vi "testControlNotOnConnectorPane.vi"() -> ()   [LabVIEW 2019, in "TestCaseTest.lvlib" / "Theory.lvlib"]
uses:
  Theory.lvlib
  TestCase/Theory/Theory.lvclass
  TestCaseTestSupport/FakeTheoryWithControlsNotOnConnectorPane.vi
  Assertion/Assertion.lvlib
  TestCaseTestSupport/TestCaseTestSupport.lvlib
panel:
  out "error out":errorcluster
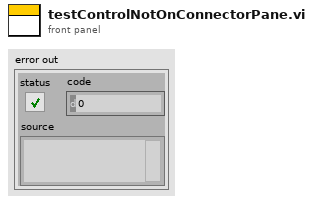
[diagram p1: front panel]
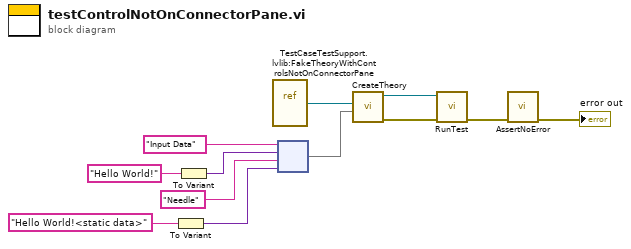
[diagram p0: block diagram]
diagram:
  n1 = To Variant(anything="Hello World!<static data>" ("key")) -> (Variant=w2:variant)
  n2 = To Variant(anything="Hello World!" ("key")) -> (Variant=w6:variant)
  n3 = vi-ref "TestCaseTestSupport.lvlib:FakeTheoryWithControlsNotOnConnectorPane.vi"() -> (w4:refnum<vi>)
  n4 = node("Input Data" ("key"), w6, "Needle" ("key"), w2) -> (w7:map{string, variant})
  n5 = call "CreateTheory.vi"("Control Data"=w7, "VI Refnum"=w4) -> ("error out"=w11:errorcluster, "Theory"=w12:refnum<class "Theory.lvclass">)  [unwired: 8 in]
  n6 = call-dynamic "RunTest.vi"("error in (no error)"=w11, "Theory in"=w12) -> ("error out"=w10:errorcluster)  [unwired: 8 in, 1 out]
  n7 = call "AssertNoError.vi"("error in (no error)"=w10) -> ("error out"=→"error out":errorcluster)  [unwired: 10 in]
